vi "Launcher App (Top Level VI).vi"() -> ()   [LabVIEW 2019]
uses:
  Architecture/Typedefs/FGV Ref. Modules Function.ctl
  Architecture/Typedefs/Enum_Module_Name.ctl
  Architecture/Typedefs/Module References.ctl
  Architecture/Typedefs/Message.ctl
  Architecture/Modules/Configuration/Main.vi
  Configuration Database/Main Database.vi
  Controller/Main Controller.vi
  Display Console/Main Display Console.vi
  UserConsole/Main User Console.vi
  Sensor Interface/Main Sensor Interface.vi
  Architecture/Architecture.lvlib
  Architecture/Modules/Configuration/Configuration.lvlib
  Configuration Database/Configuration Database.lvlib
  Controller/Controller.lvlib
  Display Console/DisplayConsole.lvlib
  Sensor Interface/Sensor Interface.lvlib
  UserConsole/UserConsole.lvlib
panel:
  out "error out":errorcluster
  in  "Loading Bar":u8(slide) caption="Loading Sensor Interface..." max=100 step=1 scale=0.0..100.0
  # "APPLICATION LAUNCHER"
  # "Juan Pérez Rodríguez"
  # "www.CtrlVIStudios.com"
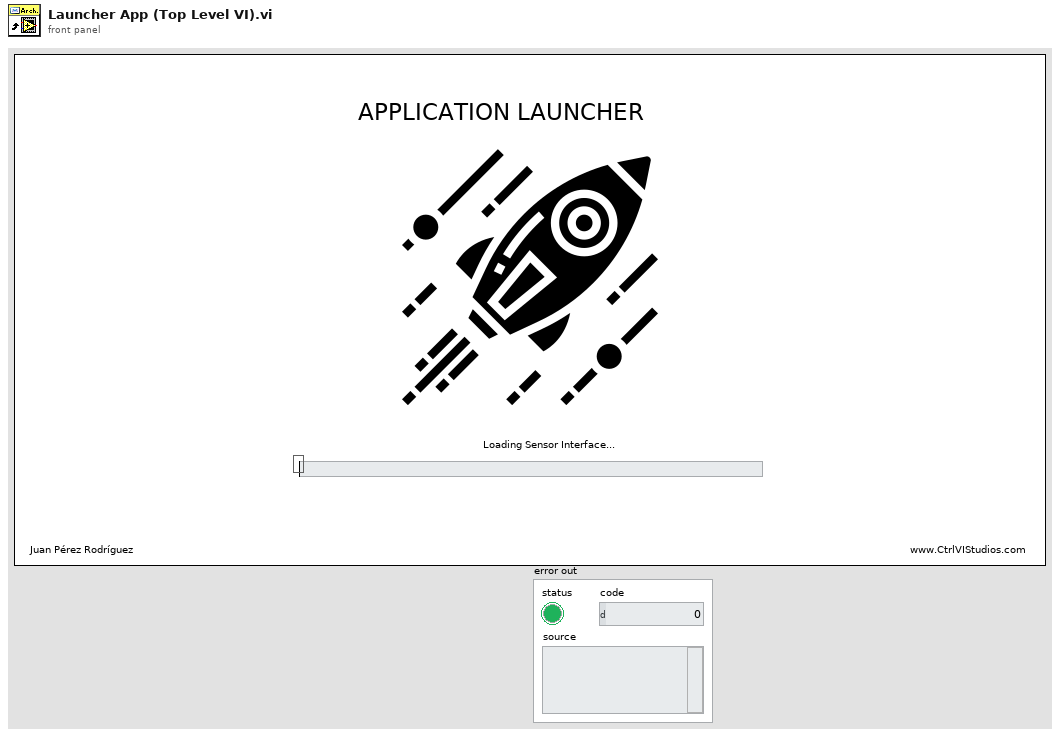
[diagram p1: front panel]
types:
  T1 = typedef "Architecture.lvlib/Enum_Module_Name.ctl" = enum16{"Configuration", "Error_Handler", "Log", "Database", "Controller", "User Console", "Display Console", "Sensor Interface"}
  T2 = cluster{"ModuleName":T1, "ShowFP":bool, "StatesTracking Enabled":bool}[]
  T3 = typedef "Architecture.lvlib/FGV Ref. Modules Function.ctl" = enum16{"Init ", "Add Module", "Get Module", "Get All", "Add Asynchronous Run Ref", "Dispose"}
  T4 = typedef "Architecture.lvlib/Module References.ctl" = cluster{"ModuleName":T1, "Queue":refnum<queue>, "user event":refnum<user-event>, "VI Refnum":refnum<vi>, "ShowFP":bool, "StatesTracking Enabled":bool}
  T5 = enum32{"invalid app kind", "Development System", "Run Time System", "Student Edition", "Embedded LabVIEW", "Evaluation", "Custom"}
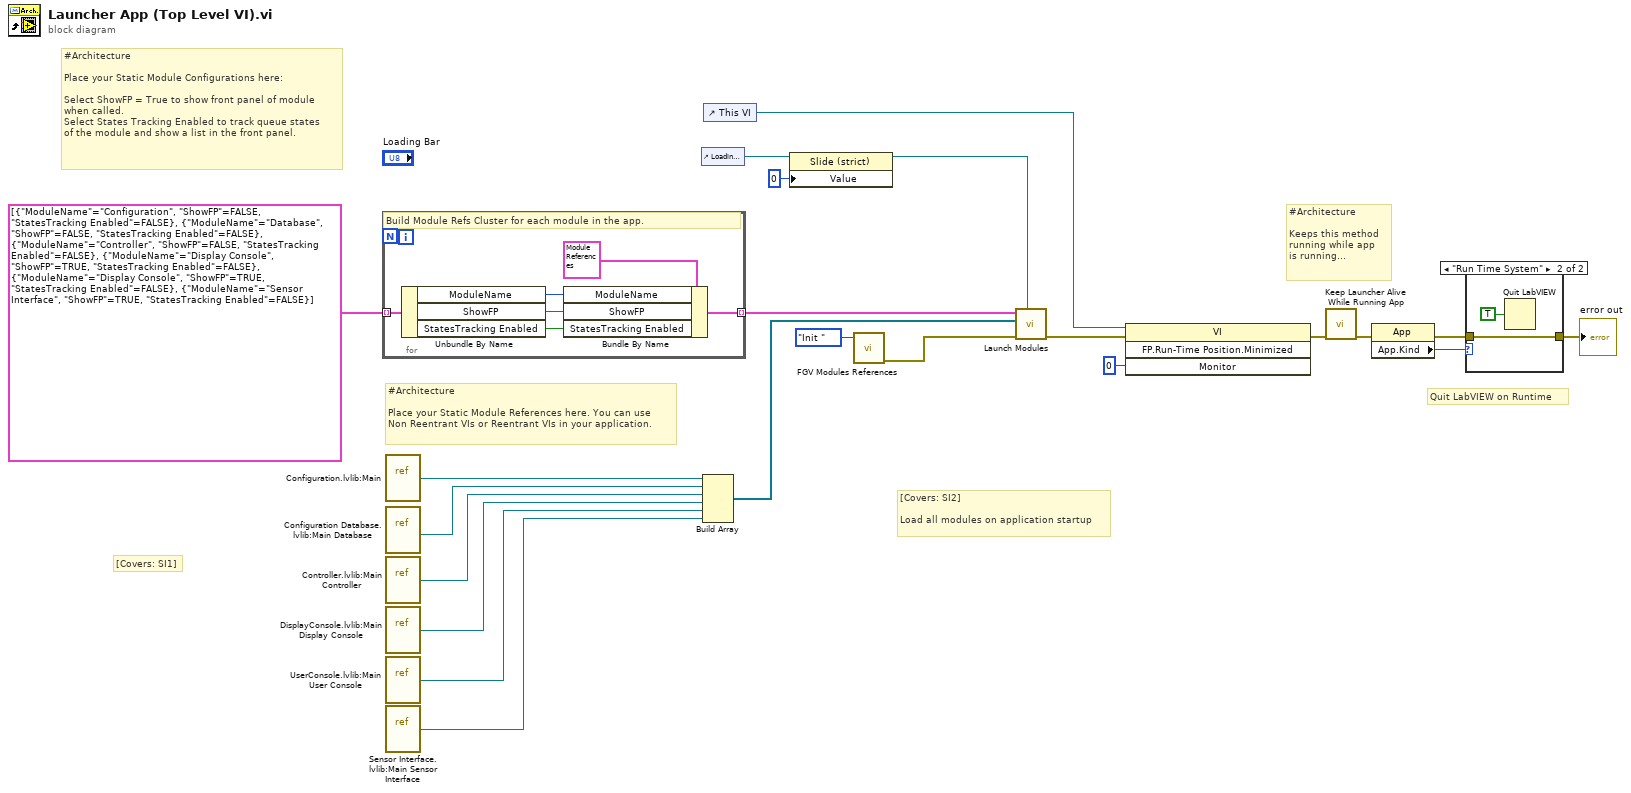
[diagram p0: block diagram]
diagram:
  # "[Covers: SI1]"
  # "[Covers: SI2]\n\nLoad all modules on application startup"
  # "#Architecture\n\nKeeps this method \nrunning while app \nis running..."
  # "Quit LabVIEW on Runtime"
  # "#Architecture\n\nPlace your Static Module References here. You can use\nNon Reentrant VIs or Reentrant VIs in your application."
  # "#Architecture\n\nPlace your Static Module Configurations here:\n\nSelect ShowFP = True to show front panel of module\nwhen called. \nSelect States Tracking Enabled to track queue states\nof the module and show a list in the front panel."
  n1 = for {
    tunnel: T2 [{"ModuleName"=enum."Configuration", "ShowFP"=FALSE, "StatesTracking Enabled"=FALSE}, {"ModuleName"=enum."Database", "ShowFP"=FALSE, "StatesTracking Enabled"=FALSE}, {"ModuleName"=enum."Controller", "ShowFP"=FALSE, "StatesTracking Enabled"=FALSE}, {"ModuleName"=enum."Display Console", "ShowFP"=TRUE, "StatesTracking Enabled"=FALSE}, {"ModuleName"=enum."Display Console", "ShowFP"=TRUE, "StatesTracking Enabled"=FALSE}, {"ModuleName"=enum."Sensor Interface", "ShowFP"=TRUE, "StatesTracking Enabled"=FALSE}] -> [w27] mode=indexing
    tunnel: [w23] -> w21 mode=indexing
    # "Build Module Refs Cluster for each module in the app."
    n2 = Unbundle By Name(w27) -> ("ModuleName"=w26:T1, "ShowFP"=w25:bool, "StatesTracking Enabled"=w24:bool)
    n3 = Bundle By Name(cluster=T4 {"ModuleName"=enum."Controller", "Queue"=refnum, "user event"=refnum, "VI Refnum"=refnum, "ShowFP"=FALSE, "StatesTracking Enabled"=FALSE} ("Module_Refs"), "ModuleName"=w26, "ShowFP"=w25, "StatesTracking Enabled"=w24) -> (w23:T4)
  }
  n4 = vi-ref "Configuration.lvlib:Main.vi"() -> (w9:refnum<vi>)
  n5 = vi-ref "Configuration Database.lvlib:Main Database.vi"() -> (w8:refnum<vi>)
  n6 = vi-ref "Controller.lvlib:Main Controller.vi"() -> (w7:refnum<vi>)
  n7 = vi-ref "DisplayConsole.lvlib:Main Display Console.vi"() -> (w6:refnum<vi>)
  n8 = vi-ref "UserConsole.lvlib:Main User Console.vi"() -> (w2:refnum<vi>)
  n9 = vi-ref "Sensor Interface.lvlib:Main Sensor Interface.vi"() -> (w1:refnum<vi>)
  n10 = control-ref of="Loading Bar"() -> (w20:refnum<vi>)
  n11 = Build Array(w9, w8, w7, w6, w2, w1) -> (w14:refnum<vi>[])
  n12 = control-ref of="This VI"() -> (w13:refnum<vi>)
  n13 = property class="Slide (strict)"(reference=w20, "Value"=u8 0) -> (reference out=w17:refnum<vi>)  [unwired: 1 in, 1 out]
  n14 = call "FGV Modules References.vi"("FGV Ref. Function In"=FGV_Ref._Modules_Function."Init ") -> ("error out"=w18:errorcluster)  [unwired: 8 in, 2 out]
  n15 = call "Launch Modules.vi"("Loading Bar Ref In"=w17, "error in (no error)"=w18, "App Modules Refs"=w14, "Modules Info In"=w21) -> ("error out"=w15:errorcluster)  [unwired: 7 in]
  n16 = invoke class="VI" method="FP.Run-Time Position.Minimized"(reference=w13, error in=w15, "Monitor"=i16 0) -> (error out=w12:errorcluster)  [unwired: 1 in, 3 out]
  n17 = call "Keep Launcher Alive While Running App.vi"("error in (no error)"=w12) -> ("error out"=w11:errorcluster)  [unwired: 10 in]
  n18 = property class="App"(error in=w11) -> (error out=w5:errorcluster, "App.Kind"=w3:T5)  [unwired: 1 in, 1 out]
  n19 = case shown="\"Run Time System\"" w3 {
    tunnel: w5 -> [w29 w31]
    tunnel: [w29 w31] -> w4
    frame Default {
    }
    frame "Run Time System" {
      n20 = Quit LabVIEW(quit? (T)=TRUE) -> ()
    }
  }
  "error out" <- w4
